vi "CCP_play_alarm_v2.vi"(5 "wav":string="error_HiPace1200.wav", 6 "time_last_in":timestamp[](array[timestamp]), 7 "audio_onoff":bool=TRUE caption="Audio\nAlarm", 9 "interval":dbl=20.0, 10 "delay":dbl=2.0, 11 "error":bool=TRUE) -> (4 "time_last_out":timestamp[](array[timestamp]))   [LabVIEW 2019]
uses:
  <vilib>/Utility/SystemLogging/NI_SystemLogging.lvlib
panel:
  # "\"time_last_in\" and \"time_last_out\" must be connected\n via Feedback Node or Shift Register in a loop that calls this sub VI."
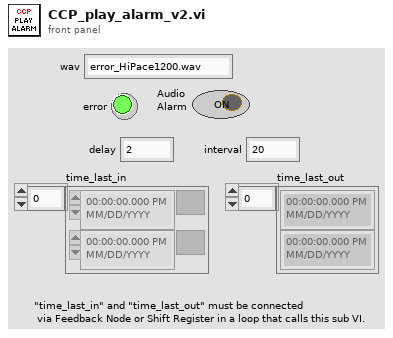
[diagram p1: front panel]
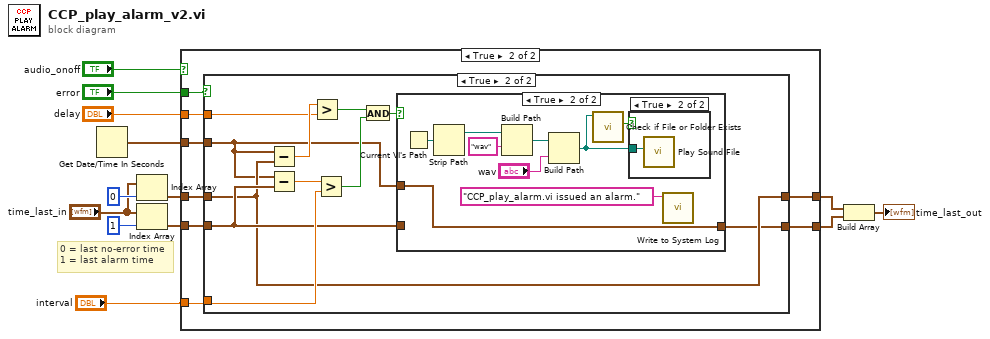
[diagram p0: block diagram]
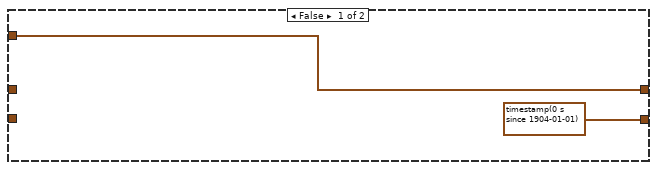
[diagram p2: hidden frame]
diagram:
  # "0 = last no-error time\n1 = last alarm time"
  n1 = Get Date/Time In Seconds() -> (seconds since 1Jan1904=w6:timestamp)
  n2 = Index Array(array="time_last_in", index=0) -> (element=w8:timestamp)
  n3 = Index Array(array="time_last_in", index=1) -> (element=w7:timestamp)
  n4 = case shown="True" "audio_onoff" {
    tunnel: "delay" -> [_ w23]
    tunnel: "interval" -> [_ w22]
    tunnel: w8 -> [_ w16]
    tunnel: w7 -> [_ w17]
    tunnel: [w14 w19] -> w5
    tunnel: w6 -> [w14 w21]
    tunnel: [timestamp(0 s since 1904-01-01) ("seconds since 1Jan1904") w18] -> w3
    tunnel: "error" -> [_ w20]
    frame False {
    }
    frame True {
      n5 = case shown="True" w20 {
        tunnel: w23 -> [_ w35]
        tunnel: w22 -> [_ w33]
        tunnel: w21 -> [w24 w26]
        tunnel: [w24 w28] -> w19
        tunnel: [w25 w27] -> w18
        tunnel: w17 -> [w25 w29]
        tunnel: w16 -> [_ w28]
        frame False {
        }
        frame True {
          n6 = Subtract(x=w26, y=w28) -> (x-y=w36:dbl)
          n7 = Subtract(x=w26, y=w29) -> (x-y=w34:dbl)
          n8 = Greater?(x=w36, y=w35) -> (0:w30:bool)
          n9 = Greater?(x=w34, y=w33) -> (0:w31:bool)
          n10 = And(x=w30, y=w31) -> (x .and. y?=w32:bool)
          n11 = case shown="True" w32 {
            tunnel: w26 -> [_ w39]
            tunnel: w29 -> [w37 _]
            tunnel: [w37 w39] -> w27
            frame False {
            }
            frame True {
              n12 = Current VI's Path() -> (path=w46:path)
              n13 = Strip Path(path=w46) -> (stripped path=w45:path)  [unwired: 1 out]
              n14 = Build Path(base path=w45, name or relative path="wav") -> (appended path=w43:path)
              n15 = Build Path(base path=w43, name or relative path="wav") -> (appended path=w41:path)
              n16 = call <vilib>:"Check if File or Folder Exists.vi"("path"=w41) -> ("file or folder exists?"=w42:bool)  [unwired: 8 in, 2 out]
              n17 = case shown="True" w42 {
                tunnel: w41 -> [_ w47]
                frame False {
                }
                frame True {
                  n18 = call <vilib>:"Play Sound File.vi"("path"=w47) -> ()  [unwired: 9 in, 2 out]
                }
              }
              n19 = call <vilib>:"Write to System Log.vi"("message"="CCP_play_alarm.vi issued an alarm.") -> ()  [unwired: 10 in, 1 out]
            }
          }
        }
      }
    }
  }
  n20 = Build Array(w5, w3) -> (→"time_last_out":timestamp[])
